vi "数据查询B.vi"(8 "Result":string, 9 "2D_Code":string, 10 "结束时间":timestamp format="%<%X\n%Y/%m/%d>T", 11 "开始时间":timestamp=timestamp(3786912000 s since 1904-01-01) format="%<%X\n%Y/%m/%d>T") -> (3 "Data":string[][](array[string]))   [LabVIEW 2014]
panel:
  out "error out":errorcluster
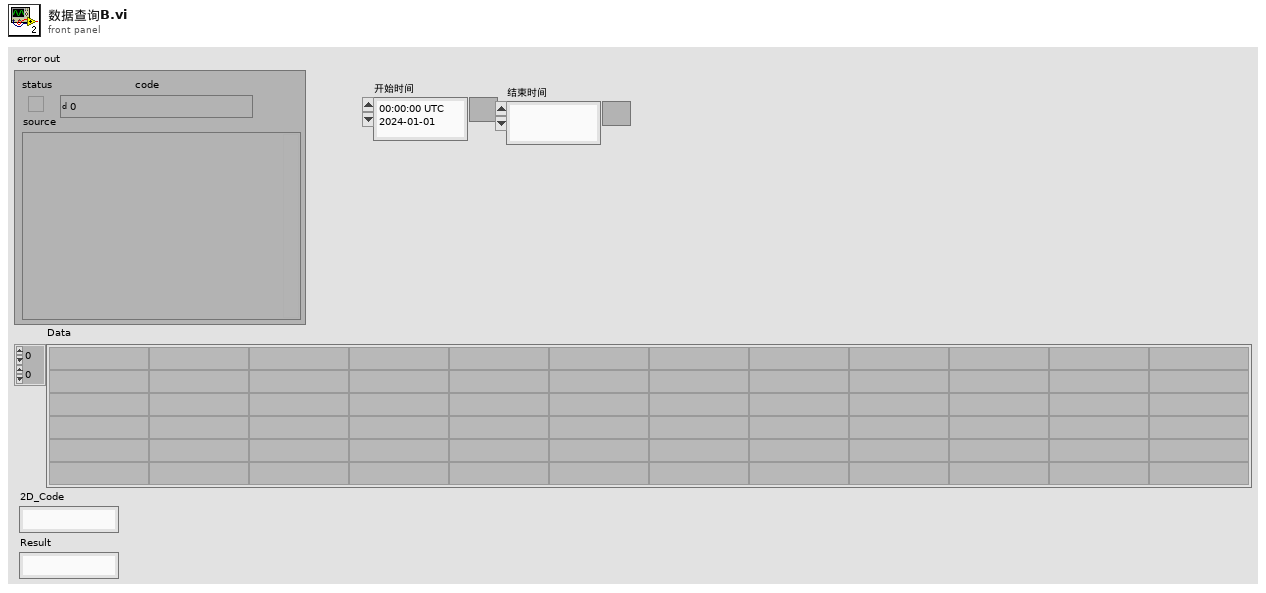
[diagram p1: front panel]
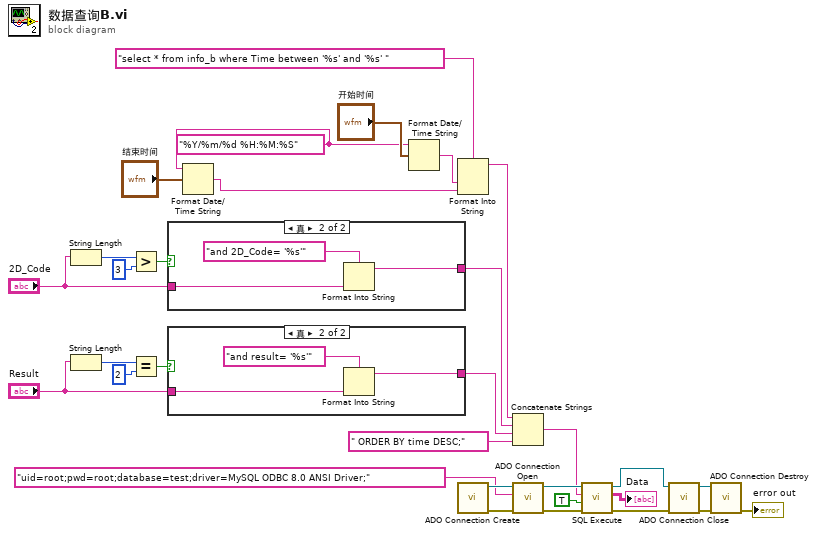
[diagram p0: block diagram]
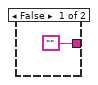
[diagram p2: hidden frame]
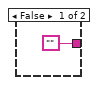
[diagram p3: hidden frame]
diagram:
  w16 = "%Y/%m/%d %H:%M:%S" ("时间格式字符串(%c)")
  n1 = String Length(string="2D_Code") -> (length=w7:i32)
  n2 = String Length(string="Result") -> (length=w3:i32)
  n3 = Greater?(x=w7, y=3) -> (0:w5:bool)
  n4 = Equal?(x=w3, y=2) -> (x = y?=w1:bool)
  n5 = case shown="真" w5 {
    tunnel: ["" w35] -> w10
    tunnel: "2D_Code" -> [_ w33]
    frame False {
    }
    frame True {
      n6 = Format Into String(format string="and 2D_Code= '%s'" ("字符串"), w33) -> (resulting string=w35:string)  [unwired: 2 in, 1 out]
    }
  }
  n7 = case shown="真" w1 {
    tunnel: ["" w39] -> w12
    tunnel: "Result" -> [_ w38]
    frame False {
    }
    frame True {
      n8 = Format Into String(format string="and result= '%s'" ("字符串"), w38) -> (resulting string=w39:string)  [unwired: 2 in, 1 out]
    }
  }
  n9 = Format Date/Time String(time format string (%c)=w16, seconds (now)="结束时间") -> (date/time string=w14:string)  [unwired: 1 in]
  n10 = Format Date/Time String(time format string (%c)=w16, seconds (now)="开始时间") -> (date/time string=w15:string)  [unwired: 1 in]
  n11 = Format Into String(format string="select * from info_b where Time between '%s' and '%s' " ("Command Text"), w15, w14) -> (resulting string=w13:string)  [unwired: 2 in, 1 out]
  n12 = call "ADO Connection Create.vi"() -> ("error out"=w30:errorcluster, "ADODB._Connection Out"=w31:refnum<k7>)  [unwired: 10 in]
  n13 = Concatenate Strings(w13, w10, w12, " ORDER BY time DESC;" ("字符串")) -> (w9:string)
  n14 = call "ADO Connection Open.vi"("error in (no error)"=w30, "ConnectionString"="uid=root;pwd=root;database=test;driver=MySQL ODBC 8.0 ANSI Driver;", "ADODB._Connection In"=w31) -> ("error out"=w28:errorcluster, "ADODB._Connection Out"=w29:refnum<k7>)  [unwired: 7 in]
  n15 = call "SQL Execute.vi"("error in (no error)"=w28, "Return Data (T)"=TRUE, "Command Text"=w9, "ADODB._Connection In"=w29) -> ("error out"=w26:errorcluster, "Data"=→"Data":string[][], "ADODB._Connection Out"=w27:refnum<k7>)  [unwired: 4 in, 1 out]
  n16 = call "ADO Connection Close.vi"("error in (no error)"=w26, "ADODB._Connection In"=w27) -> ("error out"=w24:errorcluster, "ADODB._Connection Out"=w25:refnum<k7>)  [unwired: 8 in]
  n17 = call "ADO Connection Destroy.vi"("error in (no error)"=w24, "ADODB._Connection In"=w25) -> ("error out"=→"error out":errorcluster)  [unwired: 9 in]
